vi "myRIO Tester.vi"() -> ()   [LabVIEW 2014]
uses:
  <vilib>/myRIO/Instrument Drivers/Onboard IO/DIO/vis/Write.vi
  <vilib>/myRIO/Instrument Drivers/Onboard IO/DIO/vis/Smart Open.vi
  <vilib>/Utility/error.llb/Error Cluster From Error Code.vi
  <vilib>/myRIO/Common/Instrument Driver Framework/myRIO v1.0/DIO/vis/myRIO v1.0 Write DIO.vi
panel:
  in  "Boolean":bool=TRUE
  in  "stop":bool
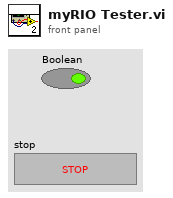
[diagram p1: front panel]
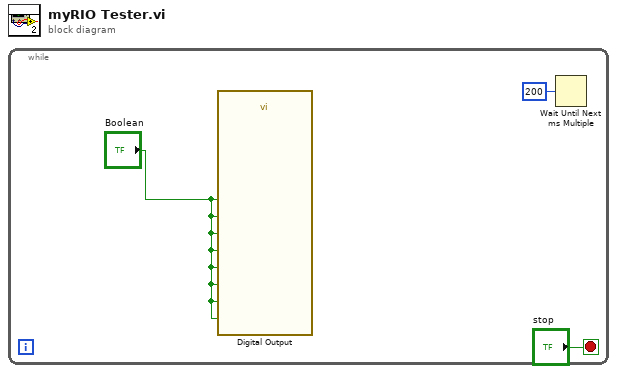
[diagram p0: block diagram]
diagram:
  n1 = while {
    stop <- "stop" stop-if-true
    n2 = call "Digital Output"("C/DIO0"="Boolean", "C/DIO1"="Boolean", "C/DIO2"="Boolean", "C/DIO3"="Boolean", "C/DIO4"="Boolean", "C/DIO5"="Boolean", "C/DIO6"="Boolean", "C/DIO7"="Boolean") -> ()  [unwired: 19 in, 1 out]
    n3 = Wait Until Next ms Multiple(millisecond multiple=u32 200) -> ()  [unwired: 1 out]
  }
